vi "Secondary Force Balance.vi"(0 "Number of MHX Baffles":dbl, 1 "MHX Tube Pitch (m)":dbl, 2 "Sec Loop Width (m)":dbl, 3 "AB Friction Factor":dbl, 4 "Sec Mass Flow (kg/s)":dbl, 5 "BC Friction Factor":dbl, 6 "Sec Loop Height (m)":dbl, 8 "NDHX Tube Length (m)":dbl, 9 "Sec Cold Density (kg/m^3)":dbl, 10 "Dctl (m)":dbl, 11 "MHX Length (m)":dbl, 12 "Shell Crossflow Area (m^2)":dbl, 13 "CEFriction Factor":dbl, 14 "Sec Cold Velocity (m/s)":dbl, 15 "Sec Hot Density (kg/m^3) in":dbl, 16 "Sec Hot Velocity (m/s)":dbl, 17 "Sec Ave Density (kg/m^3) 3":dbl, 18 "Sec NDHX Velocity (m/s)":dbl, 19 "Numeric in":dbl, 24 "Pipe Diameter (m)":dbl, 25 "NDHX Tube Diameter (m)":dbl, 26 "MHX Tube Diameter (m)":dbl, 27 "EA Friction Factor":dbl) -> (21 "Force Balance (Pa)":dbl)   [LabVIEW 2019]
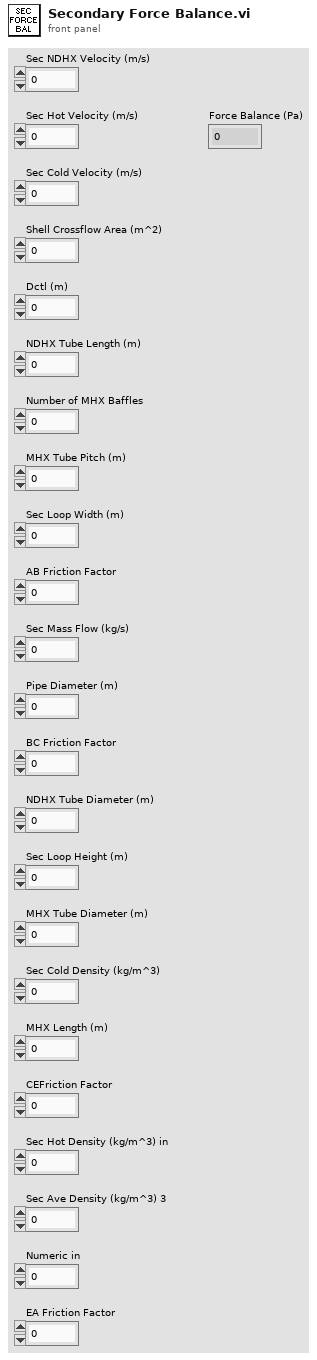
[diagram p1: front panel]
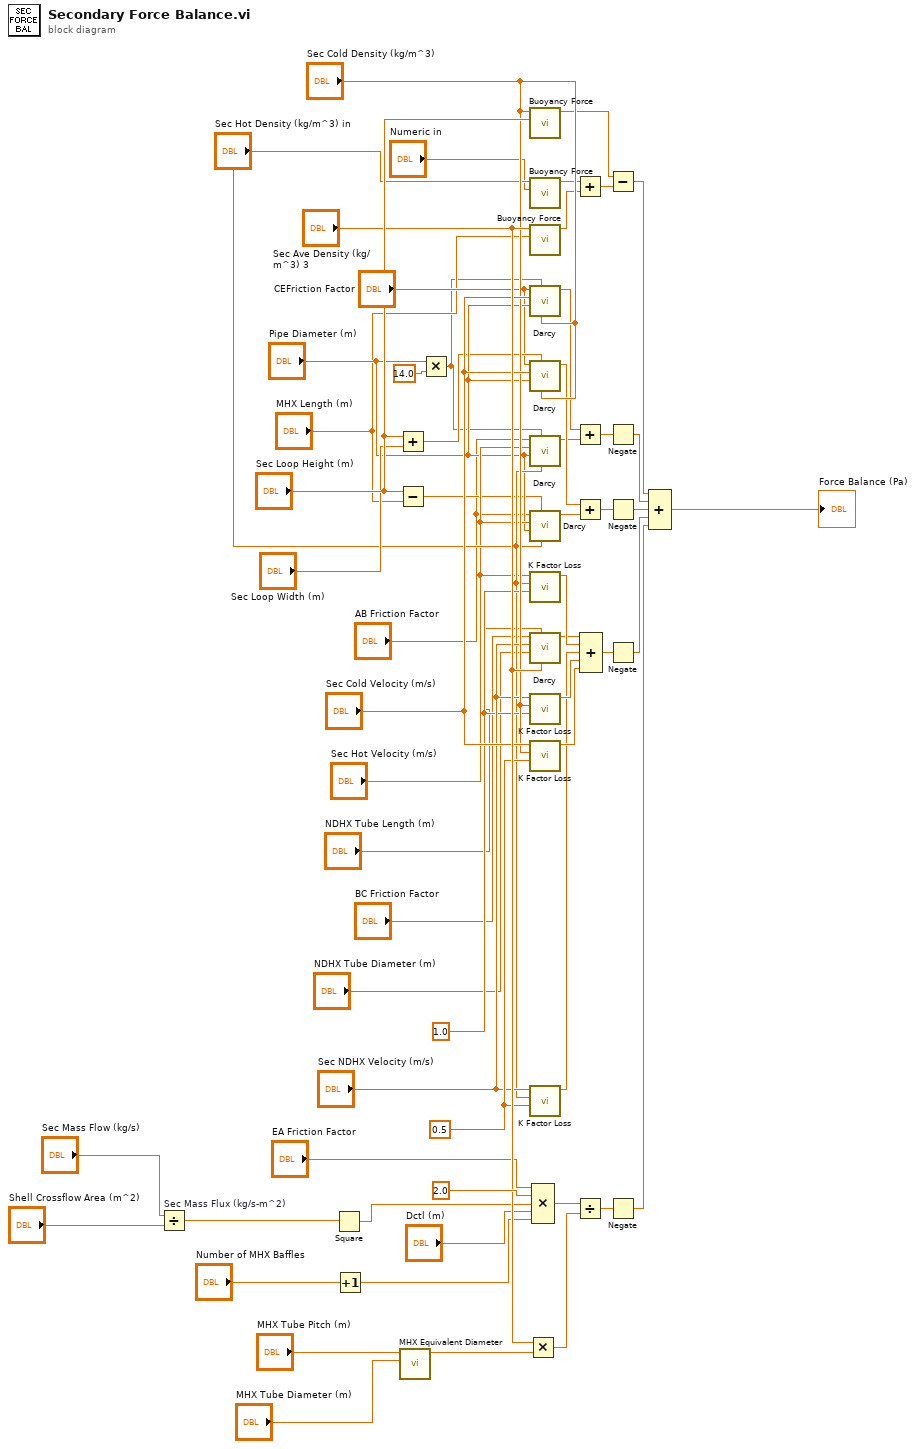
[diagram p0: block diagram]
diagram:
  w30 = 0.5 ("K")
  w28 = 1.0 ("K")
  n1 = Divide "Sec Mass Flux (kg/s-m^2)"(x="Sec Mass Flow (kg/s)", y="Shell Crossflow Area (m^2)") -> (x/y=w38:dbl)
  n2 = Square(x=w38) -> (x^2=w40:dbl)
  n3 = Increment(x="Number of MHX Baffles") -> (x+1=w43:dbl)
  n4 = Add(x="Sec Loop Height (m)", y="Sec Loop Width (m)") -> (x+y=w19:dbl)
  n5 = Subtract(x="Sec Loop Height (m)", y="MHX Length (m)") -> (x-y=w17:dbl)
  n6 = call "MHX Equivalent Diameter.vi"("MHX Tube Diameter (m)"="MHX Tube Diameter (m)", "MHX Tube Pitch (m)"="MHX Tube Pitch (m)") -> ("Numeric"=w46:dbl)  [unwired: 9 in]
  n7 = Multiply(x="Pipe Diameter (m)", y=14.0) -> (x*y=w12:dbl)
  n8 = Multiply(x="Sec Ave Density (kg/m^3) 3", y=w46) -> (x*y=w45:dbl)
  n9 = call "Buoyancy Force.vi"("Height (m)"="Sec Loop Height (m)", "Density (kg/m^3)"="Sec Cold Density (kg/m^3)") -> ("Potential (Pa)"=w5:dbl)  [unwired: 9 in]
  n10 = call "Buoyancy Force.vi"("Height (m)"="Numeric in", "Density (kg/m^3)"="Sec Hot Density (kg/m^3) in") -> ("Potential (Pa)"=w3:dbl)  [unwired: 9 in]
  n11 = call "Buoyancy Force.vi"("Height (m)"="MHX Length (m)", "Density (kg/m^3)"="Sec Ave Density (kg/m^3) 3") -> ("Potential (Pa)"=w4:dbl)  [unwired: 9 in]
  n12 = call "Darcy.vi"("Density (kg/m^3)"="Sec Cold Density (kg/m^3)", "Length (m)"=w12, "Effective Diameter (m)"="Pipe Diameter (m)", "Velocity (m/s)"="Sec Cold Velocity (m/s)", "Friction Factor"="CEFriction Factor") -> ("Loss (Pa)"=w14:dbl)  [unwired: 6 in]
  n13 = call "Darcy.vi"("Density (kg/m^3)"="Sec Cold Density (kg/m^3)", "Length (m)"=w19, "Effective Diameter (m)"="Pipe Diameter (m)", "Velocity (m/s)"="Sec Cold Velocity (m/s)", "Friction Factor"="CEFriction Factor") -> ("Loss (Pa)"=w22:dbl)  [unwired: 6 in]
  n14 = call "Darcy.vi"("Density (kg/m^3)"="Sec Hot Density (kg/m^3) in", "Length (m)"=w12, "Effective Diameter (m)"="Pipe Diameter (m)", "Velocity (m/s)"="Sec Hot Velocity (m/s)", "Friction Factor"="AB Friction Factor") -> ("Loss (Pa)"=w13:dbl)  [unwired: 6 in]
  n15 = call "Darcy.vi"("Density (kg/m^3)"="Sec Hot Density (kg/m^3) in", "Length (m)"=w17, "Effective Diameter (m)"="Pipe Diameter (m)", "Velocity (m/s)"="Sec Hot Velocity (m/s)", "Friction Factor"="AB Friction Factor") -> ("Loss (Pa)"=w21:dbl)  [unwired: 6 in]
  n16 = call "K Factor Loss.vi"("K"=w28, "Density (kg/m^3)"="Sec Hot Density (kg/m^3) in", "Velocity (m/s)"="Sec Hot Velocity (m/s)") -> ("Loss (Pa)"=w34:dbl)  [unwired: 8 in]
  n17 = call "Darcy.vi"("Density (kg/m^3)"="Sec Ave Density (kg/m^3) 3", "Length (m)"="NDHX Tube Length (m)", "Effective Diameter (m)"="NDHX Tube Diameter (m)", "Velocity (m/s)"="Sec NDHX Velocity (m/s)", "Friction Factor"="BC Friction Factor") -> ("Loss (Pa)"=w33:dbl)  [unwired: 6 in]
  n18 = call "K Factor Loss.vi"("K"=w28, "Density (kg/m^3)"="Sec Cold Density (kg/m^3)", "Velocity (m/s)"="Sec NDHX Velocity (m/s)") -> ("Loss (Pa)"=w36:dbl)  [unwired: 8 in]
  n19 = call "K Factor Loss.vi"("K"=w30, "Density (kg/m^3)"="Sec Cold Density (kg/m^3)", "Velocity (m/s)"="Sec Cold Velocity (m/s)") -> ("Loss (Pa)"=w37:dbl)  [unwired: 8 in]
  n20 = call "K Factor Loss.vi"("K"=w30, "Density (kg/m^3)"="Sec Hot Density (kg/m^3) in", "Velocity (m/s)"="Sec NDHX Velocity (m/s)") -> ("Loss (Pa)"=w35:dbl)  [unwired: 8 in]
  n21 = Compound Arithmetic op=MULTIPLY("EA Friction Factor", 2.0 ("y"), w40, "Dctl (m)", w43) -> (w44:dbl)
  n22 = Add(x=w3, y=w4) -> (x+y=w6:dbl)
  n23 = Add(x=w14, y=w13) -> (x+y=w51:dbl)
  n24 = Add(x=w22, y=w21) -> (x+y=w50:dbl)
  n25 = Divide(x=w44, y=w45) -> (x/y=w48:dbl)
  n26 = Compound Arithmetic op=ADD(w33, w34, w35, w36, w37) -> (w49:dbl)
  n27 = Subtract(x=w5, y=w6) -> (x-y=w56:dbl)
  n28 = Negate(x=w51) -> (-x=w52:dbl)
  n29 = Negate(x=w50) -> (-x=w53:dbl)
  n30 = Negate(x=w49) -> (-x=w54:dbl)
  n31 = Negate(x=w48) -> (-x=w55:dbl)
  n32 = Compound Arithmetic op=ADD(w56, w52, w53, w54, w55) -> (→"Force Balance (Pa)":dbl)
